vi "Set Speed.vi"(8 "error in (no error)":errorcluster, 10 "FlowRate":dbl caption="Flow Rate (mL/min)", 11 "KNF Settings In":T1={"VISA resource name"="", "Simulated?"=TRUE}) -> (0 "error out":errorcluster, 1 "Connection Error":bool, 3 "KNF Settings Out":T1={"VISA resource name"="", "Simulated?"=TRUE})   [LabVIEW 2021, in "KNF SIMDOS.lvlib"]
uses:
  KNF SIMDOS.lvlib
  Settings Cluster plus SIMDOS.ctl
  <vilib>/KNF LAB/Driver S/Lvlib/SIMLAB_driver_lvclass/SIMLAB_driver.lvclass
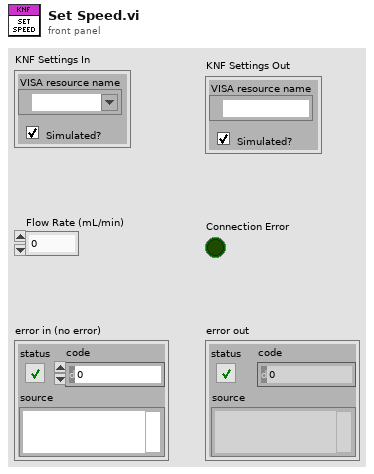
[diagram p1: front panel]
types:
  T1 = typedef "KNF SIMDOS.lvlib/Settings Cluster plus SIMDOS.ctl" = cluster{"VISA resource name":refnum<visa-resource-name>, "Simulated?":bool}
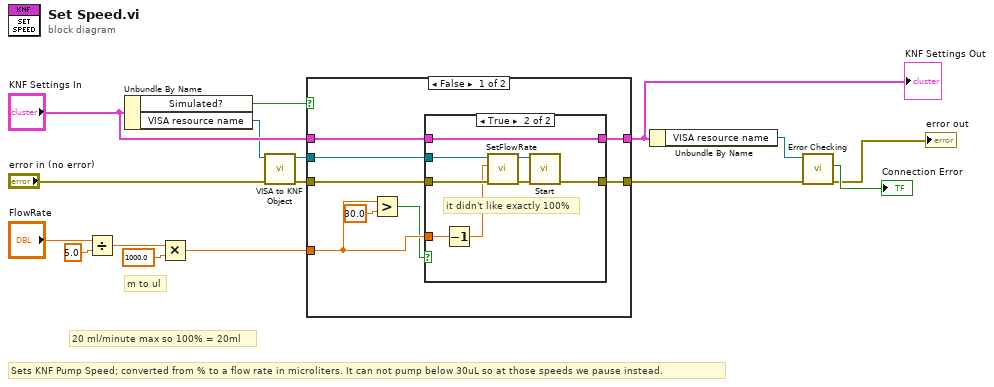
[diagram p0: block diagram]
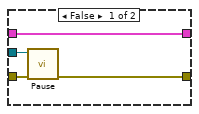
[diagram p2: hidden frame]
diagram:
  # "Sets KNF Pump Speed; converted from % to a flow rate in microliters. It can not pump below 30uL so at those speeds we pause instead."
  # "m to ul"
  # "20 ml/minute max so 100% = 20ml"
  n1 = Divide(x="FlowRate", y=5.0) -> (x/y=w6:dbl)
  n2 = Unbundle By Name("KNF Settings In") -> ("Simulated?"=w15:bool, "VISA resource name"=w12:refnum<visa-resource-name>)
  n3 = Multiply(x=w6, y=1000.0) -> (x*y=w13:dbl)
  n4 = call "VISA to KNF Object.vi"("error in (no error)"="error in (no error)", "VISA resource name"=w12) -> ("error out"=w10:errorcluster, "SIMDOS out"=w11:refnum<class "SIMLAB_driver.lvclass">)  [unwired: 8 in]
  n5 = case shown="False" w15 {
    tunnel: [w24 w38] -> w5
    tunnel: w10 -> [w22 w38]
    tunnel: [w20 w37] -> w4
    tunnel: "KNF Settings In" -> [w21 w37]
    tunnel: w11 -> [w23 _]
    tunnel: w13 -> [w19 _]
    frame False {
      n6 = Greater?(x=w19, y=30.0) -> (0:w18:bool)
      n7 = case shown="True" w18 {
        tunnel: [w26 w36] -> w24
        tunnel: w23 -> [w28 w35]
        tunnel: w22 -> [w27 w33]
        tunnel: w19 -> [_ w30]
        tunnel: w21 -> [w25 w31]
        tunnel: [w25 w31] -> w20
        frame False {
          n8 = call <vilib>:"Pause.vi"("error in (no error)"=w27, "SIMDOS in"=w28) -> ("error out"=w26:errorcluster)  [unwired: 8 in, 1 out]
        }
        frame True {
          # "it didn't like exactly 100%"
          n9 = Decrement(x=w30) -> (x-1=w29:dbl)
          n10 = call <vilib>:"SetFlowRate.vi"("error in (no error)"=w33, "FlowRate"=w29, "SIMDOS in"=w35) -> ("error out"=w32:errorcluster, "SIMDOS out"=w34:refnum<class "SIMLAB_driver.lvclass">)  [unwired: 7 in]
          n11 = call <vilib>:"Start.vi"("error in (no error)"=w32, "SIMDOS in"=w34) -> ("error out"=w36:errorcluster)  [unwired: 8 in, 1 out]
        }
      }
    }
    frame True {
    }
  }
  "KNF Settings Out" <- w4
  n12 = Unbundle By Name(w4) -> ("VISA resource name"=w3:refnum<visa-resource-name>)
  n13 = call "Error Checking.vi"("error in (no error)"=w5, "VISA resource name"=w3) -> ("error out"=→"error out":errorcluster, "Connection Error"=→"Connection Error":bool)  [unwired: 7 in, 1 out]
